vi "TDC_DAQV15_after_500MHz.vi"() -> ()   [LabVIEW 2017]
uses:
  <vilib>/Utility/file.llb/Write Delimited Spreadsheet (DBL).vi
  <vilib>/Utility/file.llb/Write Delimited Spreadsheet (I64).vi
panel:
  out "error out 2":errorcluster
  in  "display":bool=TRUE
  in  "Thresholds":u16
  in  "one key for threshold":bool
  in  "save data":bool=TRUE
  in  "RST":bool
  out "rate":dbl=7576.957857132235
  in  "Thresholds (mV)":u16[](array[numeric])=[500, 500, 500, 500, 500, 500, 500, 500]
  out "appended path 2":path=path "G:/tdc/2017/test_20230321_035424.csv"
  in  "通道数量":i32=64
  out "Cal Table":u32[](array[numeric])=[0, 0, 0, 100002, 0, 0, 0, 0, 0, 0, 0, 0, 0, 0, 0, 0, 0, 0, 0, 0, 0, 0, 0, 0, 0, 0, 0, 0, 0, 0, 0, 0]
  in  "channel for cal":i32=2
  out "single":u32 format="%08x"
  out "channel number":u64
  in  "bytes to read":i32=80
  out "Calibration Counter":i32=100000
  out "Event index":i32=97959
  out "cal":u32[](graph)
  out "error out":errorcluster
  in  "stop":bool=TRUE
  out "appended path":path=path "G:/tdc/2017/test_20230321_035424.dat"
  in  "filename":string="test"
  in  "Events":i32=110000 min=1
  in  "timeout (ms)":i32=10000
  in  "address":string="192.168.10.10"
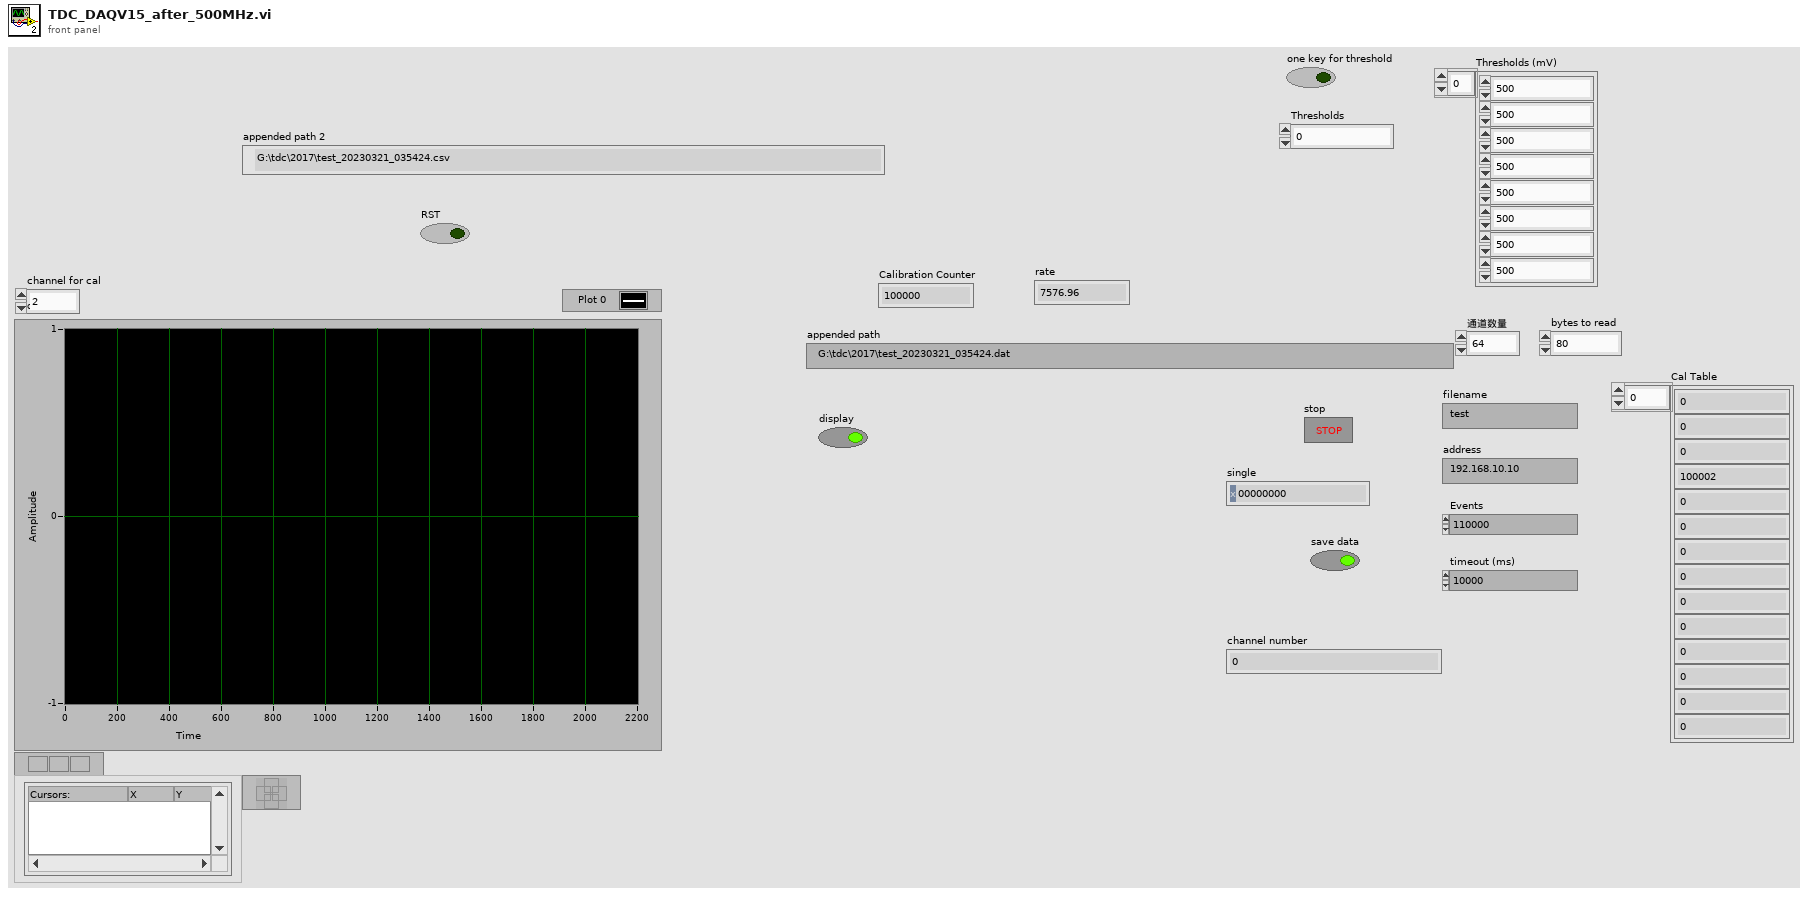
[diagram p1: front panel]
types:
  T1 = enum16{"open", "replace", "create", "open or create", "replace or create", "replace or create with confirmation"}
  T2 = enum16{"Standard", "Buffered", "CRLF", "Immediate"}
  T3 = enum16{"big-endian, network order", "native, host order", "little-endian"}
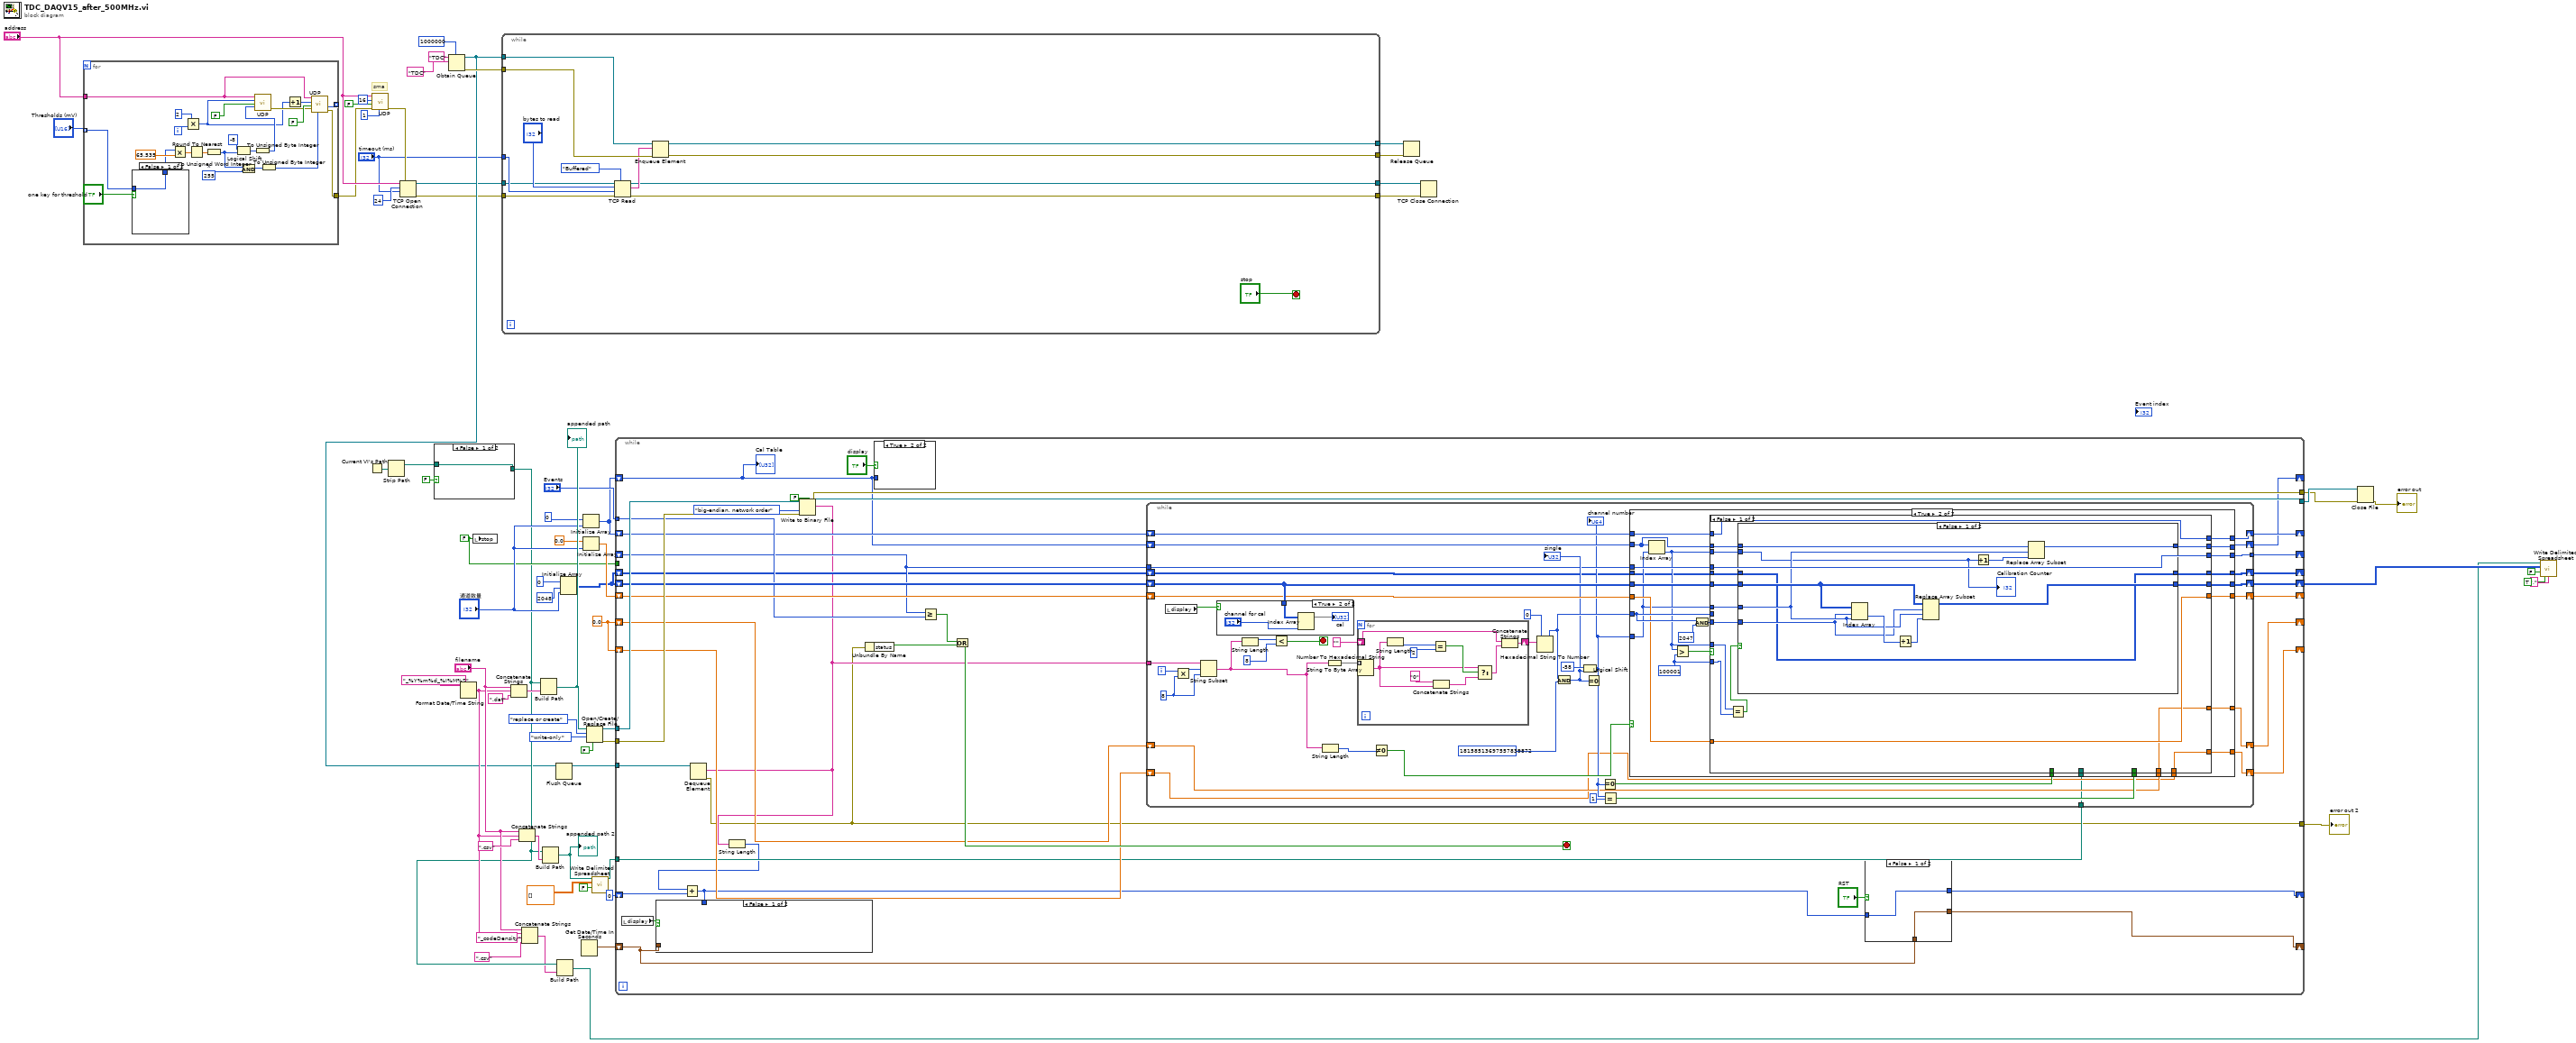
[diagram p0: block diagram]
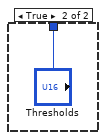
[diagram p2: hidden frame]
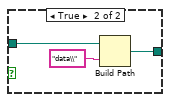
[diagram p3: hidden frame]
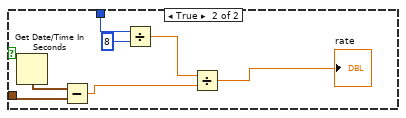
[diagram p4: hidden frame]
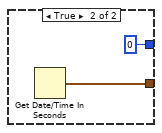
[diagram p6: hidden frame]
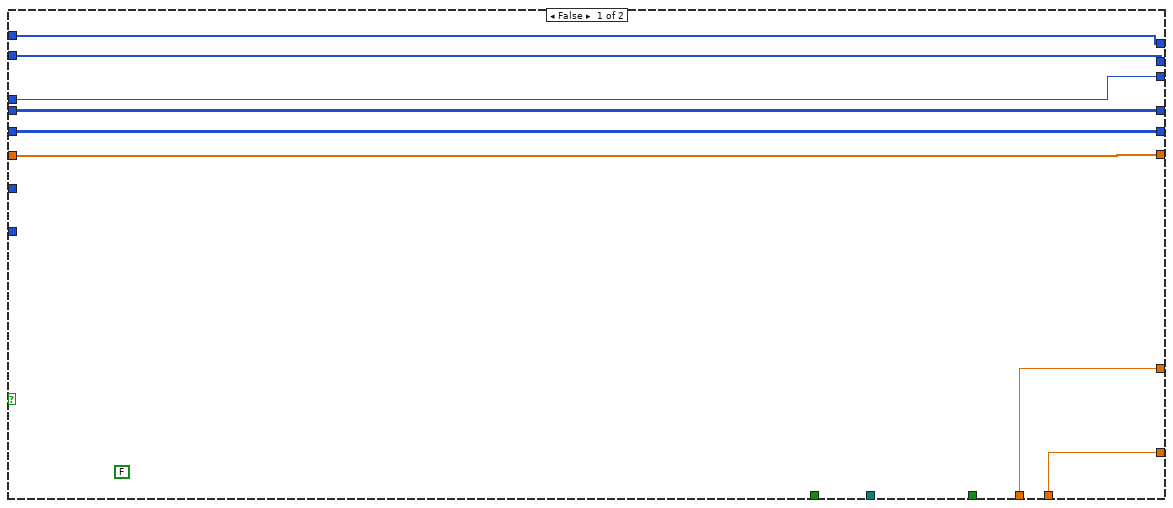
[diagram p8: hidden frame]
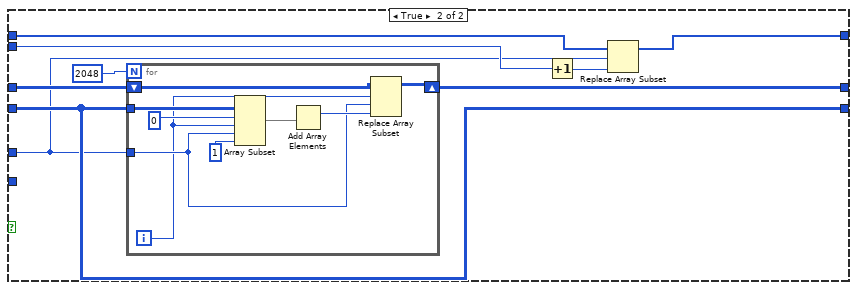
[diagram p9: hidden frame]
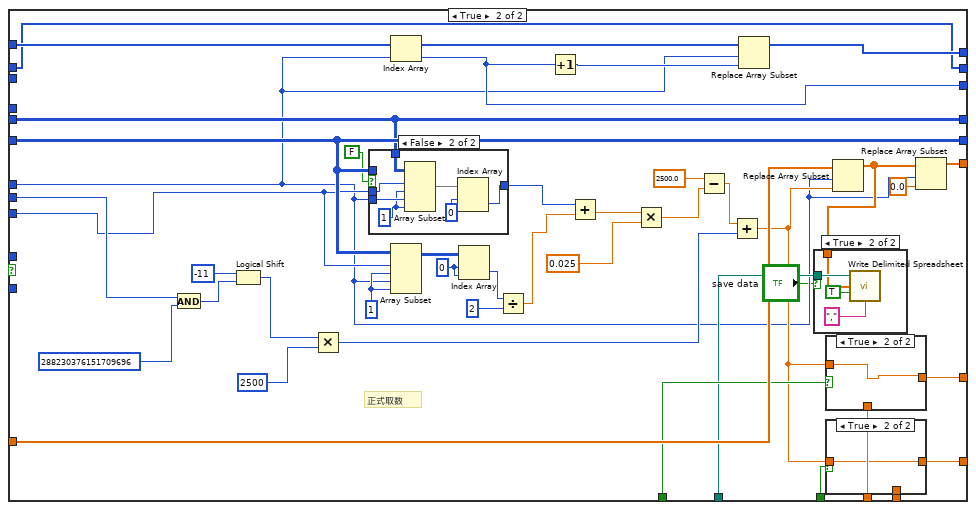
[diagram p10: hidden frame]
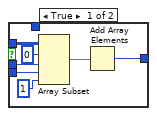
[diagram p12: hidden frame]
diagram:
  w26 = FALSE ("stop")
  w43 = 0.0
  # "sma"
  n1 = for {
    tunnel: "address" -> [w84]
    tunnel: "Thresholds (mV)" -> [w68] mode=indexing
    tunnel: [w77] -> _ mode=indexing
    tunnel: [w71] -> w30
    i -> [w90]
    w79 = u16 255  # x
    n2 = case shown="False" "one key for threshold" {
      tunnel: [w91 "Thresholds"] -> w69
      tunnel: w68 -> [w91 _]
      frame False {
      }
      frame True {
      }
    }
    n3 = Multiply(x=w69, y=65.535) -> (x*y=w87:dbl)
    n4 = Multiply(x=2, y=w90) -> (x*y=w72:i32)
    n5 = Round To Nearest(number=w87) -> (nearest integer value=w85:dbl)
    n6 = To Unsigned Word Integer(number=w85) -> (unsigned 16bit integer=w74:u16)
    n7 = Logical Shift(y=i16 -8, x=w74) -> (x << y=w81:u16)
    n8 = And(x=w74, y=w79) -> (x .and. y?=w78:u16)
    n9 = To Unsigned Byte Integer(number=w81) -> (unsigned 8bit integer=w80:u8)
    n10 = call "UDP.vi"("In"=w80, "Read (TRUE)"=FALSE, "Address"=w72, "IP address"=w84) -> ("error out"=w73:errorcluster)  [unwired: 5 in, 1 out]
    n11 = To Unsigned Byte Integer(number=w78) -> (unsigned 8bit integer=w76:u8)
    n12 = Increment(x=w72) -> (x+1=w83:i32)
    n13 = call "UDP.vi"("In"=w76, "error in (no error)"=w73, "Read (TRUE)"=FALSE, "Address"=w83, "IP address"=w84) -> ("error out"=w71:errorcluster, "Out"=w77:u8)  [unwired: 4 in]
  }
  n14 = Current VI's Path() -> (path=w61:path)
  n15 = call "UDP.vi"("In"=u8 1, "error in (no error)"=w30, "Read (TRUE)"=FALSE, "Address"=u32 16, "IP address"="address") -> ("error out"=w29:errorcluster)  [unwired: 4 in, 1 out]
  n16 = Strip Path(path=w61) -> (stripped path=w60:path)  [unwired: 1 out]
  n17 = TCP Open Connection(address="address", remote port or service name=u16 24 ("port"), timeout ms (60000)="timeout (ms)", error in (no error)=w29) -> (connection ID=w8:refnum<k5>, error out=w10:errorcluster)  [unwired: 1 in]
  n18 = case shown="False" FALSE {
    tunnel: w60 -> [w93 w95]
    tunnel: [w93 w94] -> w21
    frame False {
    }
    frame True {
      n19 = Build Path(base path=w95, name or relative path="data\\") -> (appended path=w94:path)
    }
  }
  n20 = Obtain Queue(max queue size (-1, unlimited)=1000000, name (unnamed)="TDC", element data type="TDC" ("name (unnamed)")) -> (queue out=w11:refnum<queue>, error out=w12:errorcluster)  [unwired: 2 in, 1 out]
  n21 = Format Date/Time String(time format string (%c)="_%Y%m%d_%I%M%S") -> (date/time string=w24:string)  [unwired: 2 in]
  n22 = local write "stop"(w26) -> ()
  n23 = while {
    tunnel: w11 -> [w109]
    tunnel: w12 -> [w108]
    tunnel: w10 -> [w106]
    tunnel: "timeout (ms)" -> [w105]
    tunnel: w8 -> [w104]
    tunnel: [w102] -> w7
    tunnel: [w101] -> w6
    tunnel: [w99] -> w5
    tunnel: [w98] -> w4
    stop <- "stop" stop-if-true
    n24 = TCP Read(connection ID=w104, bytes to read="bytes to read", error in (no error)=w106, 7:T2."Buffered" ("mode (standard)"), 9:w105) -> (connection ID out=w102:refnum<k5>, data out=w103:string, error out=w101:errorcluster)
    n25 = Enqueue Element(queue=w109, element=w103, error in (no error)=w108) -> (queue out=w99:refnum<queue>, error out=w98:errorcluster)  [unwired: 1 in, 1 out]
  }
  n26 = Concatenate Strings("filename", w24, ".dat") -> (w59:string)
  n27 = Concatenate Strings("filename", w24, ".csv") -> (w45:string)
  n28 = Concatenate Strings("filename", w24, "_codeDensity" ("string"), ".csv") -> (w20:string)
  n29 = Build Path(base path=w21, name or relative path=w59) -> (appended path=w58:path)
  "appended path" <- w58
  n30 = Build Path(base path=w21, name or relative path=w45) -> (appended path=w40:path)
  "appended path 2" <- w40
  n31 = Flush Queue(queue=w11) -> (queue out=w1:refnum<queue>)  [unwired: 1 in, 2 out]
  n32 = Build Path(base path=w21, name or relative path=w20) -> (appended path=w17:path)
  n33 = Initialize Array(u32 0 ("element"), 2048 ("dimension size"), "通道数量") -> (w42:u32[][])
  n34 = Get Date/Time In Seconds() -> (seconds since 1Jan1904=w33:timestamp)
  n35 = Initialize Array(u32 0 ("element"), "通道数量") -> (w44:u32[])
  n36 = Initialize Array(0.0, "通道数量") -> (w50:dbl[])
  n37 = Open/Create/Replace File(file path (use dialog)=w58, operation (0:open)=T1."replace or create", access (0:read/write)=enum16{"read/write", "read-only", "write-only"}."write-only", disable buffering (F)=FALSE) -> (refnum out=w63:refnum<file>, error out=w62:errorcluster)  [unwired: 2 in, 1 out]
  n38 = call-poly <vilib>:"Write Delimited Spreadsheet.vi"("file path (dialog if empty)"=w40, "2D data"=dbl[][] [], "append to file? (new file:F)"=FALSE) -> ("new file path (Not A Path if cancelled)"=w39:path)  [unwired: 11 in, 1 out]
  n39 = while {
    tunnel: w63 -> [w147]
    tunnel: w62 -> [w148]
    tunnel: [w111] -> w3
    tunnel: [w146] -> w55
    tunnel: [w145] -> w54
    shift-right: [w141] -> w18
    shift-left: w42 -> [w142]
    shift-right: [w125] -> _
    shift-left: w50 -> [w140]
    tunnel: "Events" -> [w137]
    shift-right: [w136] -> _
    shift-left: w44 -> [w135]
    shift-right: [w134] -> _
    shift-left: _ -> [w133]
    shift-right: [w132] -> _
    shift-left: w44 -> [w114]
    shift-right: [w131] -> _
    shift-left: w43 -> [w128]
    shift-right: [w130] -> _
    shift-left: w43 -> [w129]
    shift-right: [w117] -> _
    shift-left: w42 -> [w127]
    tunnel: w39 -> [w126]
    shift-right: [w121] -> _
    shift-left: 0 -> [w124]
    shift-right: [w119] -> _
    shift-left: w33 -> [w118]
    tunnel: w26 -> [_]
    tunnel: w1 -> [w113]
    stop <- w139 stop-if-true
    n40 = local read "display"() -> (w115:bool)
    n41 = Dequeue Element(queue=w113) -> (element=w112:string, error out=w111:errorcluster)  [unwired: 2 in, 2 out]
    n42 = String Length(string=w112) -> (length=w123:i32)
    n43 = Add(x=w123, y=w124) -> (x+y=w122:i32)
    n44 = case shown="False" w115 {
      tunnel: w122 -> [_ w150]
      tunnel: w118 -> [_ w149]
      frame False {
      }
      frame True {
        n45 = Get Date/Time In Seconds() -> (seconds since 1Jan1904=w154:timestamp)
        n46 = Subtract(x=w154, y=w149) -> (x-y=w153:dbl)
        n47 = Divide(x=w150, y=8) -> (x/y=w152:dbl)
        n48 = Divide(x=w152, y=w153) -> (x/y=→"rate":dbl)
      }
    }
    n49 = Write to Binary File(file (use dialog)=w147, data=w112, error in=w148, 5:FALSE ("prepend array or string size? (T)"), 9:T3."big-endian, network order" ("byte order (0:big-endian, network order)")) -> (refnum out=w146:refnum<file>, error out=w145:errorcluster)  [unwired: 1 in, 1 out]
    n50 = Unbundle By Name(w111) -> ("status"=w110:bool)
    n51 = case shown="True" "display" {
      tunnel: w114 -> [_ _]
      frame False {
      }
      frame True {
      }
    }
    n52 = Greater Or Equal?(x=w133, y=w137) -> (x >= y?=w138:bool)
    n53 = Or(x=w138, y=w110) -> (x .or. y?=w139:bool)
    n54 = while {
      tunnel: w112 -> [w195]
      shift-right: [w191] -> w141
      shift-left: w142 -> [w189]
      shift-right: [w187] -> w125
      shift-left: w140 -> [w188]
      shift-right: [w181] -> w136
      shift-left: w135 -> [w180]
      tunnel: [w179] -> w134
      tunnel: w133 -> [w178]
      shift-right: [w176] -> w132
      shift-left: w114 -> [w177]
      shift-right: [w168] -> w131
      shift-left: w128 -> [w166]
      shift-right: [w164] -> w130
      shift-left: w129 -> [w165]
      tunnel: w126 -> [w162]
      shift-right: [w161] -> w117
      shift-left: w127 -> [w163]
      i -> [w193]
      stop <- w184 stop-if-true
      w192 = 8 ("length (rest)")
      n55 = local read "display"() -> (w160:bool)
      n56 = Multiply(x=w193, y=w192) -> (x*y=w194:i32)
      n57 = String Subset(string=w195, offset (0)=w194, length (rest)=w192) -> (substring=w175:string)
      n58 = case shown="True" w160 {
        tunnel: w189 -> [_ w202]
        frame False {
        }
        frame True {
          n59 = Index Array(array=w202, index (col)="channel for cal") -> (element=→"cal":u32[])  [unwired: 1 in]
        }
      }
      n60 = String Length(string=w175) -> (length=w186:i32)
      n61 = Less?(x=w186, y=8) -> (x < y?=w184:bool)
      n62 = String Length(string=w175) -> (length=w173:i32)
      n63 = String To Byte Array(string=w175) -> (unsigned byte array=w198:u8[])
      n64 = for {
        shift-right: [w355] -> w197
        shift-left: "" ("format string") -> [w352]
        tunnel: w198 -> [w356] mode=indexing
        n65 = Number To Hexadecimal String(2:w356) -> (0:w348:string)  [unwired: 1 in]
        n66 = String Length(string=w348) -> (length=w354:i32)
        n67 = Equal?(x=w354, y=2) -> (x = y?=w351:bool)
        n68 = Concatenate Strings("0" ("format string"), w348) -> (w350:string)
        n69 = Select(t=w348, s=w351, f=w350) -> (s? t:f=w347:string)
        n70 = Concatenate Strings(w352, w347) -> (w355:string)
      }
      n71 = Not Equal To 0?(x=w173) -> (x != 0?=w172:bool)
      n72 = Hexadecimal String To Number(string=w197, default (0uL)=u64 0 ("default (0 U32)")) -> (number=w190:u64)  [unwired: 1 in, 1 out]
      n73 = And(x=w190, y=u64 18158513697557839872 ("port")) -> (x .and. y?=w182:u64)
      "single" <- w182
      n74 = Logical Shift(y=i16 -58, x=w182) -> (x << y=w171:u64)
      "channel number" <- w171
      n75 = Equal To 0?(x=w182) -> ()  [unwired: 1 out]
      n76 = Equal To 0?(x=w171) -> (x = 0?=w169:bool)
      n77 = Equal?(x=w171, y=u64 1) -> (x = y?=w167:bool)
      n78 = case shown="True" w172 {
        tunnel: w190 -> [_ w236]
        tunnel: w178 -> [w207 w226]
        tunnel: w189 -> [w210 w235]
        tunnel: [w210 w234] -> w191
        tunnel: [w209 w231] -> w187
        tunnel: w188 -> [w209 w230]
        tunnel: w171 -> [_ w225]
        tunnel: w180 -> [w208 w229]
        tunnel: [w208 w228] -> w181
        tunnel: [w207 w227] -> w179
        tunnel: w177 -> [w206 w224]
        tunnel: [w206 w223] -> w176
        tunnel: w169 -> [_ w222]
        tunnel: w166 -> [w205 w221]
        tunnel: [w205 w220] -> w168
        tunnel: w167 -> [_ w219]
        tunnel: w165 -> [w204 w218]
        tunnel: [w204 w217] -> w164
        tunnel: w163 -> [w203 w214]
        tunnel: [w203 w213] -> w161
        tunnel: w162 -> [_ w212]
        frame False {
          (unwired) FALSE
        }
        frame True {
          w215 = 100001 ("y")
          n79 = Index Array(array=w224, index=w225) -> (element=w216:u32)
          n80 = Greater?(x=w216, y=w215) -> (0:w211:bool)
          n81 = And(x=w236, y=u64 2047 ("port")) -> (x .and. y?=w232:u64)
          n82 = case shown="False" w211 {
            tunnel: w236 -> [_ w324]
            tunnel: w235 -> [w253 w306]
            tunnel: [w252 w306] -> w234
            tunnel: w232 -> [w244 w304]
            tunnel: [w251 w287] -> w231
            tunnel: w230 -> [w251 w313]
            tunnel: w226 -> [w249 _]
            tunnel: w225 -> [w247 w285]
            tunnel: w229 -> [w250 w312]
            tunnel: [w250 w311] -> w228
            tunnel: [w249 w309] -> w227
            tunnel: w216 -> [w245 _]
            tunnel: w224 -> [w248 w308]
            tunnel: [w246 w308] -> w223
            tunnel: w222 -> [_ w300]
            tunnel: w221 -> [w243 w299]
            tunnel: [w243 w298] -> w220
            tunnel: w219 -> [_ w297]
            tunnel: w218 -> [w242 w296]
            tunnel: [w242 w295] -> w217
            tunnel: w216 -> [w240 _]
            tunnel: w215 -> [w237 _]
            tunnel: w214 -> [w239 w289]
            tunnel: [w238 w289] -> w213
            tunnel: w212 -> [_ w288]
            frame False {
              n83 = Equal?(x=w240, y=w237) -> (x = y?=w241:bool)
              n84 = case shown="False" w241 {
                tunnel: w253 -> [w264 w270]
                tunnel: [w262 w270] -> w252
                tunnel: w248 -> [w260 w268]
                tunnel: w247 -> [w259 w265]
                tunnel: [w257 w267] -> w246
                tunnel: w245 -> [w256 w266]
                tunnel: w244 -> [w255 _]
                tunnel: w239 -> [w254 w272]
                tunnel: [w254 w271] -> w238
                frame False {
                  n85 = Index Array(array=w264, index (row)=w255, index (col)=w259) -> (element=w263:u32)
                  n86 = Increment(x=w263) -> (x+1=w261:u32)
                  n87 = Replace Array Subset(array=w264, new element=w261, index (row)=w255, index (col)=w259) -> (w262:u32[][])
                  n88 = Increment(x=w256) -> (x+1=w258:u32)
                  n89 = Replace Array Subset(array=w260, new element=w258, index=w259) -> (w257:u32[])
                  "Calibration Counter" <- w256
                }
                frame True {
                  n90 = for {
                    N: 2048 -> [_]
                    tunnel: w270 -> [w282]
                    tunnel: w265 -> [w275]
                    shift-right: [w277] -> w271
                    shift-left: w272 -> [w278]
                    i -> [w274]
                    n91 = Array Subset(array=w282, index (row)=0 ("索引"), length (row)=w274, index (col)=w275, length (col)=1 ("长度")) -> (w279:u32[][])
                    n92 = Add Array Elements(numeric array=w279) -> (sum=w276:u32)
                    n93 = Replace Array Subset(array=w278, new element=w276, index (row)=w274, index (col)=w275) -> (w277:u32[][])
                  }
                  n94 = Increment(x=w266) -> (x+1=w269:u32)
                  n95 = Replace Array Subset(array=w268, new element=w269, index=w265) -> (w267:u32[])
                }
              }
            }
            frame True {
              w302 = 0 ("索引 (行)")
              w305 = 1 ("长度")
              # "正式取数"
              n96 = And(x=w324, y=u64 288230376151709696 ("port")) -> (x .and. y?=w321:u64)
              n97 = Logical Shift(y=i16 -11, x=w321) -> (x << y=w316:u64)
              n98 = Multiply(x=w316, y=u64 2500) -> (x*y=w314:u64)
              n99 = case shown="False" FALSE {
                tunnel: [w330 w337] -> w319
                tunnel: w306 -> [w333 _]
                tunnel: w285 -> [w332 w342]
                tunnel: w304 -> [w331 w340]
                tunnel: w289 -> [_ w341]
                frame True {
                  n100 = Array Subset(array=w333, index (row)=0 ("索引"), length (row)=w331, index (col)=w332, length (col)=1 ("长度")) -> (w334:u32[][])
                  n101 = Add Array Elements(numeric array=w334) -> (sum=w330:u32)
                }
                frame False {
                  w336 = 0 ("index (row)")
                  w339 = 1 ("长度")
                  n102 = Array Subset(array=w341, index (row)=w340, length (row)=w339, index (col)=w342, length (col)=w339) -> (w338:u32[][])
                  n103 = Index Array(array=w338, index (row)=w336, index (col)=w336) -> (element=w337:u32)
                }
              }
              n104 = Index Array(array=w312, index=w285) -> (element=w309:u32)
              n105 = Array Subset(array=w306, index (row)=w304, length (row)=w305, index (col)=w285, length (col)=w305) -> (w303:u32[][])
              n106 = Index Array(array=w303, index (row)=w302, index (col)=w302) -> (element=w301:u32)
              n107 = Divide(x=w301, y=u32 2) -> (x/y=w307:dbl)
              n108 = Increment(x=w309) -> (x+1=w310:u32)
              n109 = Add(x=w319, y=w307) -> (x+y=w318:dbl)
              n110 = Multiply(x=w318, y=0.025) -> (x*y=w292:dbl)
              n111 = Subtract(x=2500.0, y=w292) -> (x-y=w291:dbl)
              n112 = Add(x=w291, y=w314) -> (x+y=w294:dbl)
              n113 = Replace Array Subset(array=w312, new element=w310, index=w285) -> (w311:u32[])
              n114 = case shown="True" w300 {
                tunnel: w294 -> [_ w346]
                tunnel: [w345 w346] -> w298
                tunnel: w299 -> [w345 _]
                frame False {
                }
                frame True {
                }
              }
              n115 = case shown="True" w297 {
                tunnel: [w343 w344] -> w295
                tunnel: w296 -> [w343 _]
                tunnel: w294 -> [_ w344]
                frame False {
                }
                frame True {
                }
              }
              n116 = Replace Array Subset(array=w313, new element=w294, index=w285) -> (w286:dbl[])
              n117 = case shown="True" "save data" {
                tunnel: w288 -> [_ w328]
                tunnel: w286 -> [_ w325]
                frame False {
                }
                frame True {
                  n118 = call-poly <vilib>:"Write Delimited Spreadsheet.vi"("file path (dialog if empty)"=w328, "1D data"=w325, "append to file? (new file:F)"=TRUE, "delimiter (\\t)"="," ("delimiter (\\t)")) -> ()  [unwired: 10 in, 2 out]
                }
              }
              n119 = Replace Array Subset(array=w286, new element=0.0 ("new element/subarray"), index=w285) -> (w287:dbl[])
            }
          }
        }
      }
    }
    n120 = case shown="False" "RST" {
      tunnel: w122 -> [w157 _]
      tunnel: [w157 0] -> w121
      tunnel: [w156 w158] -> w119
      tunnel: w118 -> [w156 _]
      frame False {
      }
      frame True {
        n121 = Get Date/Time In Seconds() -> (seconds since 1Jan1904=w158:timestamp)
      }
    }
    "Cal Table" <- w114
  }
  "error out 2" <- w3
  n122 = Release Queue(queue=w5, error in (no error)=w4) -> ()  [unwired: 1 in, 3 out]
  n123 = TCP Close Connection(connection ID=w7, error in (no error)=w6) -> ()  [unwired: 1 in, 2 out]
  n124 = Close File(refnum=w55, error in=w54) -> (error out=→"error out":errorcluster)  [unwired: 1 out]
  n125 = call-poly <vilib>:"Write Delimited Spreadsheet.vi"("file path (dialog if empty)"=w17, "2D data"=w18, "append to file? (new file:F)"=FALSE, "transpose? (no:F)"=TRUE, "delimiter (\\t)"="," ("delimiter (\\t)")) -> ()  [unwired: 9 in, 2 out]
